vi "createSubList_Scopes.vi"(11 "showAll array":refnum<vi>[](array[refnum])) -> (3 "String":string)   [LabVIEW 2013]
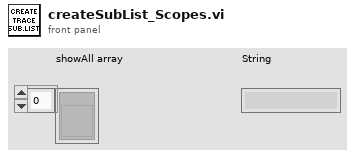
[diagram p1: front panel]
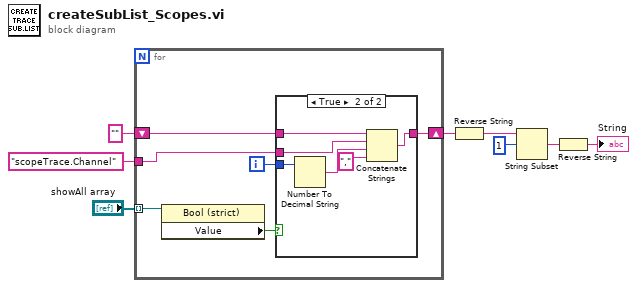
[diagram p0: block diagram]
diagram:
  n1 = for {
    shift-right: [w14] -> w2
    shift-left: "" -> [w13]
    tunnel: "scopeTrace.Channel" -> [w12]
    tunnel: "showAll array" -> [w10] mode=indexing
    i -> [w11]
    n2 = property class="Bool (strict)"(reference=w10) -> ("Value"=w9:bool)  [unwired: 1 in, 2 out]
    n3 = case shown="True" w9 {
      tunnel: [w15 w21] -> w14
      tunnel: w13 -> [w15 w20]
      tunnel: w12 -> [_ w19]
      tunnel: w11 -> [_ w16]
      frame False {
      }
      frame True {
        n4 = Number To Decimal String(number=w16) -> (decimal integer string=w18:string)  [unwired: 1 in]
        n5 = Concatenate Strings(w20, w19, w18, "," ("string")) -> (w21:string)
      }
    }
  }
  n6 = Reverse String(1:w2) -> (0:w3:string)
  n7 = String Subset(string=w3, offset (0)=1) -> (substring=w5:string)  [unwired: 1 in]
  n8 = Reverse String(1:w5) -> (0:→"String":string)
